vi "003LockerCombo.vi"() -> ()   [LabVIEW 2010]
panel:
  out "Can Open?":bool
  in  "#4":i32
  in  "#3":i32
  in  "#2":i32
  in  "#1":i32
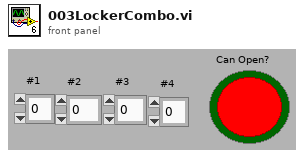
[diagram p1: front panel]
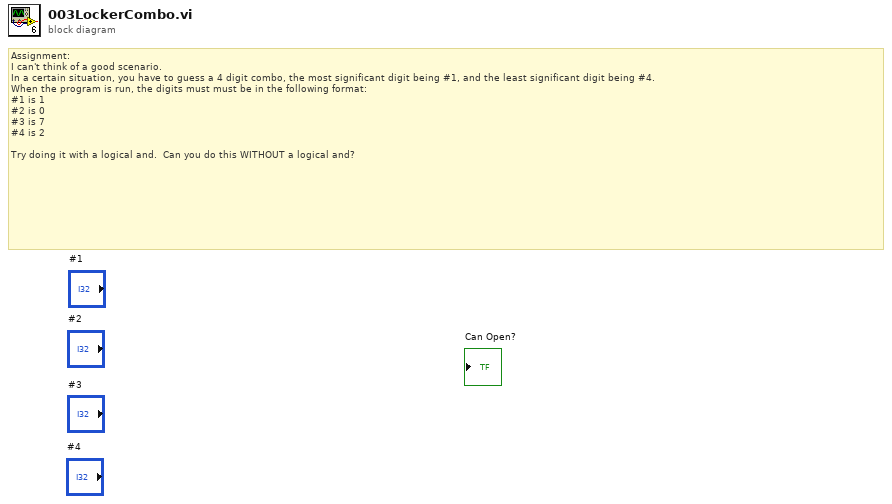
[diagram p0: block diagram]
diagram:
  # "Assignment:\nI can't think of a good scenario.\nIn a certain situation, you have to guess a 4 digit combo, the most significant digit being #1, and the least significant digit being #4.\nWhen the program is run, the digits must must be in the following format:\n#1 is 1\n#2 is 0\n#3 is 7\n#4 is 2\n\nTry doing it with a logical and.  Can you do this WITHOUT a logical and?"
